vi "Needle_measurement.vi"() -> ()   [LabVIEW 2016]
uses:
  <instrlib>/Keithley 24XX/Public/Data/Read (Statistical).vi
  <instrlib>/Keithley 24XX/Public/Data/Read (Single Point).vi
  <instrlib>/Keithley 24XX/Keithley 24XX.lvlib
panel:
  out "Voltage":sgl
  out "Current*Resistance":sgl
  in  "Enable Voltage Auto Range (T:Enable)":bool
  in  "Single measurement?":bool
  in  "Statistical Operation (0: Mean)":u16(ring) items=["Mean", "Standard Deviation", "Maximum", "Minimum", "Peak to Peak"]
  in  "Sample Count (10)":i32=10
  in  "Source Mode  (0: Voltage)":u16(ring) items=["Voltage", "Current"]
  in  "Compliance  Level (uA)":dbl=0.1
  in  "Output Level (0)":dbl
  in  "Voltage Manual Range (1.0)":dbl=1.0
  out "Resistance":sgl
  out "Current":sgl
  in  "Serial Configuration":T1={"Baud Rate"=9600, "Parity"=0, "Data Bits"=8, "Stop Bits"=10, "Flow Control"=0} {"Flow Control" items=["None", "XON/XOFF", "RTS/CTS", "XON/XOFF & RTS/CTS", "DTR/DSR", "XON/XOFF & DTR/DSR"]; "Stop Bits" items=["1.0"=10, "1.5"=15, "2.0"=20]; "Data Bits" items=["7"=7, "8"=8]; "Parity" items=["None", "Odd", "Even", "Mark", "Space"]; "Baud Rate" items=["300"=300, "600"=600, "1200"=1200, "2400"=2400, "4800"=4800, "9600"=9600, "19200"=19200]}
  in  "VISA resource name":refnum<visa-resource-name>
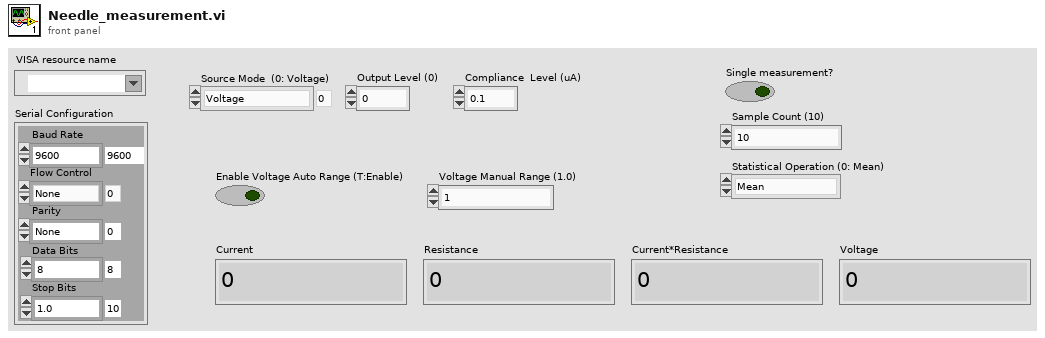
[diagram p1: front panel]
types:
  T1 = cluster{"Baud Rate":u32, "Parity":u16, "Data Bits":u16, "Stop Bits":u16, "Flow Control":u16}
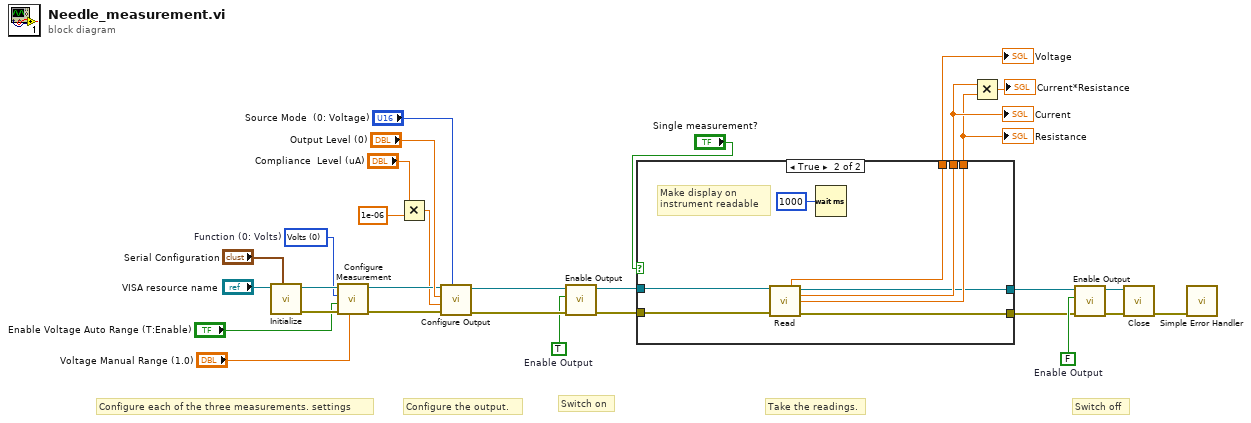
[diagram p0: block diagram]
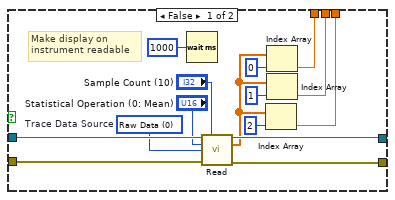
[diagram p2: hidden frame]
diagram:
  w13 = TRUE  # Enable Output
  w23 = FALSE  # Enable Output
  w25 = u16 0 items=["Volts", "Current", "Resistance"]  # Function (0: Volts)
  # "Switch on"
  # "Switch off"
  # "Take the readings."
  # "Configure the output."
  # "Configure each of the three measurements. settings"
  n1 = call <instrlib>:"Initialize.vi"("Serial Configuration"="Serial Configuration", "VISA resource name"="VISA resource name") -> ("error out"=w26:errorcluster, "VISA resource name out"=w27:refnum<visa-resource-name>)  [unwired: 8 in]
  n2 = call <instrlib>:"Configure Measurement.vi"("Manual Range (1.0)"="Voltage Manual Range (1.0)", "error in (no error)"=w26, "Enable Auto Range (T:Enable)"="Enable Voltage Auto Range (T:Enable)", "Function (0: Volts)"=w25, "VISA resource name"=w27) -> ("error out"=w10:errorcluster, "VISA resource name out"=w11:refnum<visa-resource-name>)  [unwired: 5 in]
  n3 = Multiply(x="Compliance  Level (uA)", y=1e-06) -> (x*y=w7:dbl)
  n4 = call <instrlib>:"Configure Output.vi"("Source Mode  (0: Voltage)"="Source Mode  (0: Voltage)", "error in (no error)"=w10, "Compliance  Level (0.1)"=w7, "Output Level (0)"="Output Level (0)", "VISA resource name"=w11) -> ("error out"=w14:errorcluster, "VISA resource name out"=w15:refnum<visa-resource-name>)  [unwired: 5 in]
  n5 = call <instrlib>:"Enable Output.vi"("error in (no error)"=w14, "Enable Output (T: Enable)"=w13, "VISA resource name"=w15) -> ("error out"=w17:errorcluster, "VISA resource name out"=w16:refnum<visa-resource-name>)  [unwired: 7 in]
  n6 = case shown="True" "Single measurement?" {
    tunnel: [w36 w53] -> w3
    tunnel: [w35 w52] -> w2
    tunnel: [w44 w51] -> w19
    tunnel: [w42 w50] -> w18
    tunnel: w17 -> [w45 w49]
    tunnel: w16 -> [w43 w48]
    tunnel: [w32 w47] -> w1
    frame False {
      w37 = u16 0 items=["Raw Data", "Math Data", "Limit Data"]  # Trace Data Source
      # "Make display on instrument readable"
      n7 = Wait (ms)(milliseconds to wait=u32 1000) -> ()  [unwired: 1 out]
      n8 = call-poly <instrlib>:"Read.vi"("VISA resource name"=w43, "Sample Count (2)"="Sample Count (10)", "Statistical Operation (0: Mean)"="Statistical Operation (0: Mean)", "Trace Data Source (0: Raw Data)"=w37, "error in (no error)"=w45) -> ("VISA resource name out"=w42:refnum<visa-resource-name>, "Statistical Operation Results"=w33:dbl[], "error out"=w44:errorcluster)  [unwired: 8 in]
      n9 = Index Array(array=w33, index=2) -> (element=w35:dbl)
      n10 = Index Array(array=w33, index=0) -> (element=w32:dbl)
      n11 = Index Array(array=w33, index=1) -> (element=w36:dbl)
    }
    frame True {
      # "Make display on instrument readable"
      n12 = call-poly <instrlib>:"Read.vi"("VISA resource name"=w48, "error in (no error)"=w49) -> ("Voltage"=w47:sgl, "VISA resource name out"=w50:refnum<visa-resource-name>, "Current"=w53:sgl, "Resistance"=w52:sgl, "error out"=w51:errorcluster)  [unwired: 7 in, 2 out]
      n13 = Wait (ms)(milliseconds to wait=u32 1000) -> ()  [unwired: 1 out]
    }
  }
  "Current" <- w3
  "Resistance" <- w2
  "Voltage" <- w1
  n14 = Multiply(x=w3, y=w2) -> (x*y=→"Current*Resistance":dbl)
  n15 = call <instrlib>:"Enable Output.vi"("error in (no error)"=w19, "Enable Output (T: Enable)"=w23, "VISA resource name"=w18) -> ("error out"=w20:errorcluster, "VISA resource name out"=w21:refnum<visa-resource-name>)  [unwired: 7 in]
  n16 = call <instrlib>:"Close.vi"("error in (no error)"=w20, "VISA resource name"=w21) -> ("error out"=w30:errorcluster)  [unwired: 9 in]
  n17 = call <vilib>:"Simple Error Handler.vi"("error in (no error)"=w30) -> ()  [unwired: 4 in, 5 out]
